vi "TCP_wrapper.vi"(11 "Cluster":cluster{i32, string}) -> ()   [LabVIEW 2019, in "Protocols.lvlib"]
uses:
  Protocols.lvlib
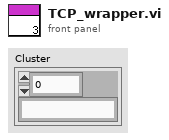
[diagram p1: front panel]
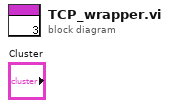
[diagram p0: block diagram]
diagram:
